vi "LabVIEW Measurement UI - Stop & Close.vi"(8 "error in":errorcluster, 10 "UI Subpanel":refnum<vi>, 11 "Measurement Client Wrapper in":refnum<class "Measurement Client Wrapper.lvclass">) -> (0 "error out":errorcluster, 3 "Measurement Client Wrapper":refnum<class "Measurement Client Wrapper.lvclass">)   [LabVIEW 2020, in "Measurement Client Wrapper.lvclass"]
uses:
  Measurement Client Wrapper.lvclass
  Measurement Client Wrapper.lvclass/Measurement Client Wrapper.ctl
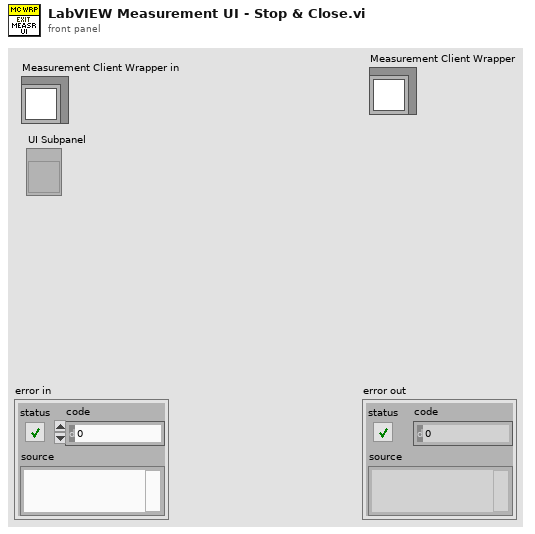
[diagram p1: front panel]
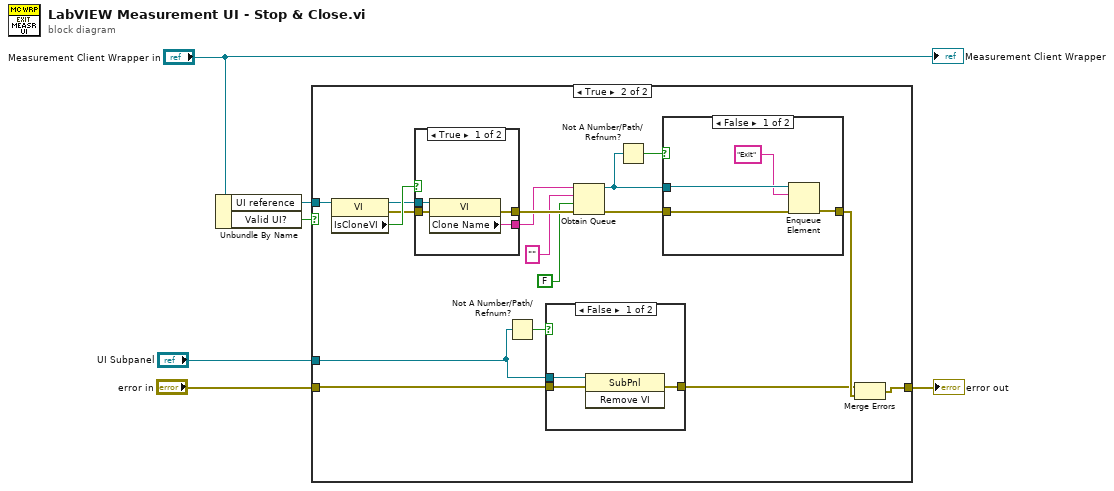
[diagram p0: block diagram]
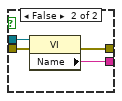
[diagram p5: hidden frame]
diagram:
  n1 = Unbundle By Name("Measurement Client Wrapper in") -> ("UI reference"=w6:refnum<vi>, "Valid UI?"=w1:bool)
  n2 = case shown="True" w1 {
    tunnel: w6 -> [_ w13]
    tunnel: [w7 w12] -> w4
    tunnel: "error in" -> [w7 w11]
    tunnel: "UI Subpanel" -> [_ w8]
    frame False {
    }
    frame True {
      n3 = property class="VI"(reference=w13) -> (reference out=w22:refnum<vi>, error out=w23:errorcluster, "IsCloneVI"=w24:bool)  [unwired: 1 in]
      n4 = case shown="True" w24 {
        tunnel: w23 -> [w37 w41]
        tunnel: w22 -> [w36 w40]
        tunnel: [w35 w39] -> w20
        tunnel: [w34 w38] -> w21
        frame True {
          n5 = property class="VI"(reference=w36, error in=w37) -> (error out=w34:errorcluster, "Clone Name"=w35:string)  [unwired: 1 out]
        }
        frame False {
          n6 = property class="VI"(reference=w40, error in=w41) -> (error out=w38:errorcluster, "Name"=w39:string)  [unwired: 1 out]
        }
      }
      n7 = Not A Number/Path/Refnum?(number/path/refnum=w8) -> (NaN/Path/Refnum?=w9:bool)
      n8 = case shown="False" w9 {
        tunnel: w8 -> [w27 _]
        tunnel: [w26 w28] -> w10
        tunnel: w11 -> [w25 w28]
        frame False {
          n9 = invoke class="SubPnl" method="Remove VI"(reference=w27, error in=w25) -> (error out=w26:errorcluster)  [unwired: 1 in, 2 out]
        }
        frame True {
        }
      }
      n10 = Obtain Queue(name (unnamed)=w20, element data type="", create if not found? (T)=FALSE, error in (no error)=w21) -> (queue out=w15:refnum<queue>, error out=w16:errorcluster)  [unwired: 1 in, 1 out]
      n11 = Not A Number/Path/Refnum?(number/path/refnum=w15) -> (NaN/Path/Refnum?=w17:bool)
      n12 = case shown="False" w17 {
        tunnel: w16 -> [w31 w33]
        tunnel: w15 -> [w32 _]
        tunnel: [w30 w33] -> w14
        frame False {
          n13 = Enqueue Element(queue=w32, element="Exit", error in (no error)=w31) -> (error out=w30:errorcluster)  [unwired: 1 in, 2 out]
        }
        frame True {
        }
      }
      n14 = Merge Errors(w10, w14) -> (w12:errorcluster)
    }
  }
  "error out" <- w4
  "Measurement Client Wrapper" <- "Measurement Client Wrapper in"
